vi "Timed Write to Hardware.vi"(7 "Triggers Valid":bool, 8 "error in":errorcluster, 9 "Trigger Values":dbl[](array[numeric]), 10 "Values":dbl[](array[numeric]), 11 "Execution Unit in":refnum<class "Execution Unit.lvclass">) -> (0 "error out":errorcluster, 1 "Trigger Values out":dbl[](array[numeric]), 2 "Values out":dbl[](array[numeric]), 3 "Execution Unit out":refnum<class "Execution Unit.lvclass">)   [LabVIEW 2020, in "Ballard MIL-STD-1553 Engine.lvlib" / "Custom Device.lvlib"]
uses:
  Custom Device.lvlib
  Interfaces/Execution Unit/Execution Unit.lvclass
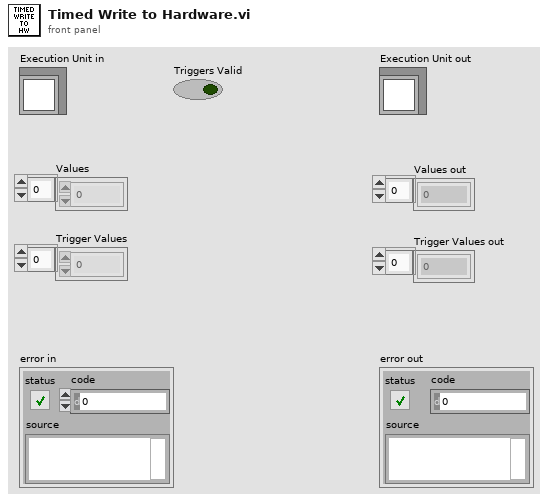
[diagram p1: front panel]
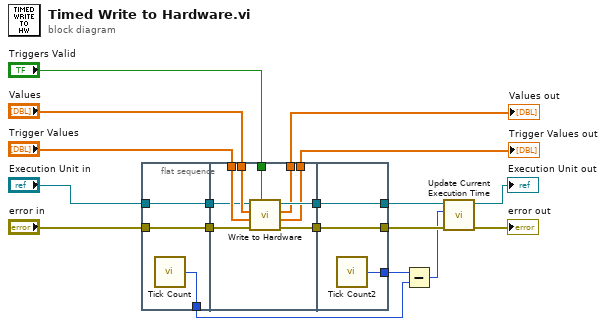
[diagram p0: block diagram]
diagram:
  n1 = flat-sequence {
    tunnel: "Execution Unit in" -> [w19]
    tunnel: "error in" -> [w20]
    tunnel: [w20] -> w8
    tunnel: [w19] -> w7
    tunnel: [w18] -> w4
    tunnel: "Triggers Valid" -> [w29]
    tunnel: "Trigger Values" -> [w27]
    tunnel: "Values" -> [w25]
    tunnel: [w28] -> w10
    tunnel: [w24] -> w9
    tunnel: w8 -> [w26]
    tunnel: w7 -> [w23]
    tunnel: [w22] -> w2
    tunnel: [w21] -> w1
    tunnel: [w31] -> w12
    tunnel: [w32] -> w16
    tunnel: w10 -> [w32]
    tunnel: w9 -> [w31]
    tunnel: [w30] -> w5
    frame #0 {
      n2 = call "Tick Count"() -> ("Tick Count(uSec)"=w18:u32)
    }
    frame #1 {
      n3 = call-dynamic "Write to Hardware.vi"("Valid Triggers"=w29, "error in (no error)"=w26, "Trigger Values"=w27, "Values in"=w25, "Execution Unit in"=w23) -> ("error out"=w28:errorcluster, "Trigger Values out"=w21:dbl[], "Values out"=w22:dbl[], "Execution Unit out"=w24:refnum<class "Execution Unit.lvclass">)  [unwired: 3 in]
    }
    frame #2 {
      n4 = call "Tick Count2"() -> ("Tick Count(uSec)"=w30:u32)
    }
  }
  n5 = Subtract(x=w5, y=w4) -> (x-y=w3:u32)
  n6 = call-dynamic "Update Current Execution Time.vi"("Current Execution Time (us)"=w3, "Execution Unit in"=w12) -> ("Execution Unit out"=→"Execution Unit out":refnum<class "Execution Unit.lvclass">)  [unwired: 8 in, 1 out]
  "error out" <- w16
  "Values out" <- w2
  "Trigger Values out" <- w1
